vi "Write ctlVal.vi"(8 "error in (no error)":errorcluster, 10 "ctlVal":T1, 11 "Meerstetter TEC in":refnum<class "Meerstetter TEC.lvclass">) -> (0 "error out":errorcluster, 3 "Meerstetter TEC out":refnum<class "Meerstetter TEC.lvclass">)   [LabVIEW 2014, in "Meerstetter Lib.lvlib" / "Meerstetter TEC.lvclass"]
uses:
  Meerstetter TEC.lvclass
  Controls/Ctl Method.ctl
  Meerstetter TEC.lvclass/Meerstetter TEC.ctl
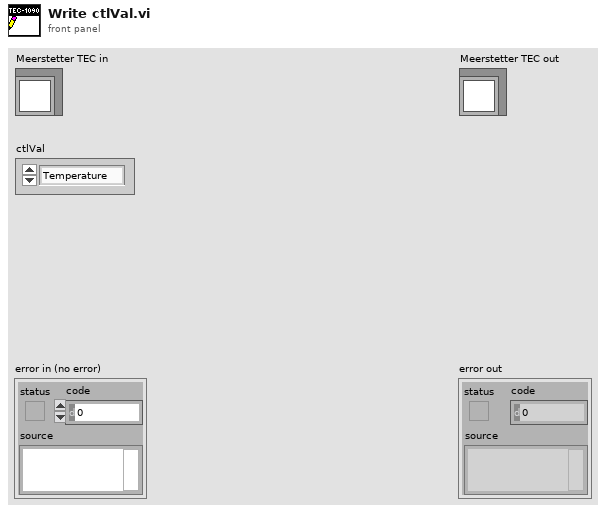
[diagram p1: front panel]
types:
  T1 = typedef "Meerstetter Lib.lvlib/Meerstetter TEC.lvclass/Ctl Method.ctl" = enum16{"Temperature", "Power"}
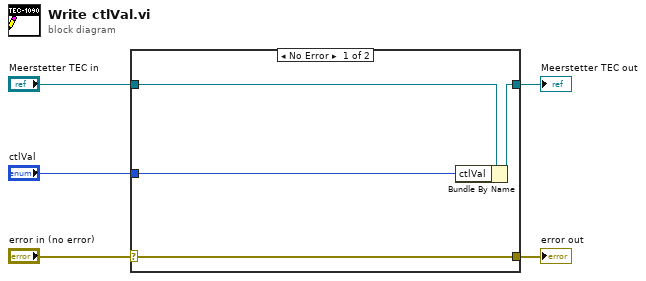
[diagram p0: block diagram]
diagram:
  n1 = case shown="No Error" "error in (no error)" {
    selector: "error in (no error)" -> [w9 w10]
    tunnel: [w9 w10] -> w4
    tunnel: [w7 w11] -> w2
    tunnel: "Meerstetter TEC in" -> [w8 w11]
    tunnel: "ctlVal" -> [w6 _]
    frame No Error {
      n2 = Bundle By Name(cluster=w8, "ctlVal"=w6) -> (w7:refnum<class "Meerstetter TEC.lvclass">)
    }
    frame Error {
    }
  }
  "error out" <- w4
  "Meerstetter TEC out" <- w2
